vi "DataChange.vi"(9 "值":string[](array[string])=["名称", "文本程序", "关键字"], 10 "键名":string, 11 "段名":string) -> ()   [LabVIEW 2018]
uses:
  <vilib>/Utility/config.llb/Write Key (String).vi
  <vilib>/Utility/config.llb/NI_LVConfig.lvlib
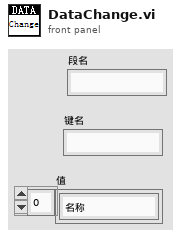
[diagram p1: front panel]
types:
  T1 = typedef "NI_LVConfig.lvlib/Config Data RefNum.ctl" = refnum<k1>
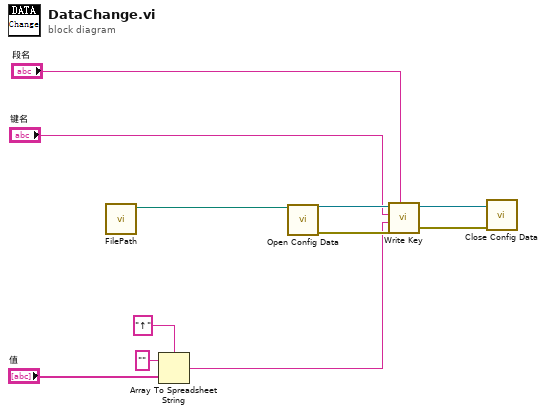
[diagram p0: block diagram]
diagram:
  n1 = call "FilePath.vi"() -> ("添加的路径"=w1:path)  [unwired: 11 in]
  n2 = Array To Spreadsheet String(delimiter (Tab)="↑" ("分隔符(Tab)"), array="值", 3:"" ("格式字符串")) -> (spreadsheet string=w6:string)
  n3 = call <vilib>:"Open Config Data.vi"("configuration file path"=w1) -> ("error out"=w10:errorcluster, "refnum"=w11:T1)  [unwired: 8 in, 1 out]
  n4 = call-poly <vilib>:"Write Key.vi"("section"="段名", "error in (no error)"=w10, "value"=w6, "key"="键名", "refnum"=w11) -> ("error out"=w2:errorcluster, "refnum out"=w3:T1)  [unwired: 4 in, 1 out]
  n5 = call <vilib>:"Close Config Data.vi"("error in (no error)"=w2, "refnum"=w3) -> ()  [unwired: 8 in, 2 out]
